vi "csv-from-string-timestamps.vi"(7 "LabVIEW Web Service Request":refnum<class "Web Request.lvclass">, 9 "format":string, 10 "end":string, 11 "start":string) -> (3 "Data":string)   [LabVIEW 2017]
uses:
  <vilib>/wsapi/Web Request.lvclass
  private/GlobalVariable.vi
panel:
  # "Use the Web Service Request input terminal to call the VIs on the Web Services palette. Do not remove it from the connector pane unless you don't need access to the palette."
  # "Each additional control wired to the connector pane will be available as an input in the URL. To include an indicator in terminal-mode output (the default setting), it must also be wired to the connector pane."
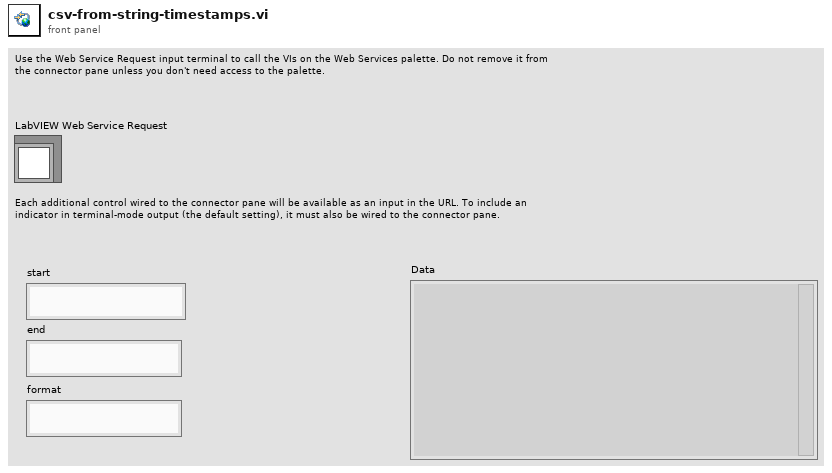
[diagram p1: front panel]
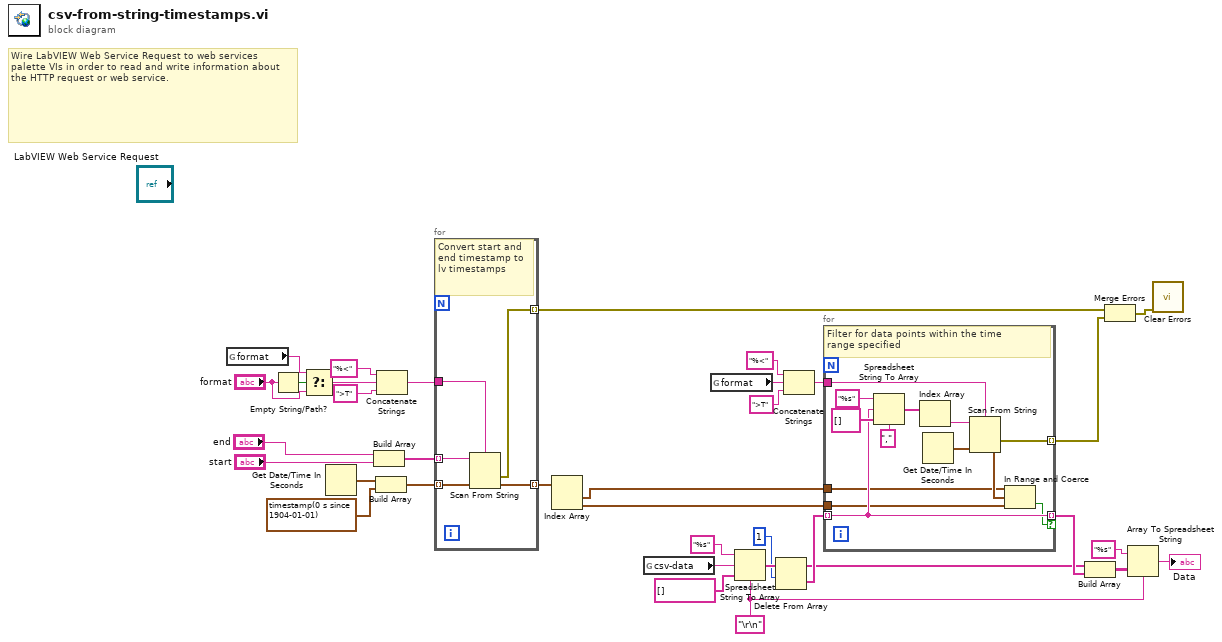
[diagram p0: block diagram]
diagram:
  w9 = "\r\n" ("format string")
  # "Wire LabVIEW Web Service Request to web services palette VIs in order to read and write information about the HTTP request or web service."
  n1 = global read "GlobalVariable.vi" "format"() -> (w4:string)
  n2 = Empty String/Path?(string/path="format") -> (empty?=w7:bool)
  n3 = Select(t=w4, s=w7, f="format") -> (s? t:f=w5:string)
  n4 = Get Date/Time In Seconds() -> (seconds since 1Jan1904=w31:timestamp)
  n5 = Build Array("end", "start") -> (w33:string[])
  n6 = Build Array(w31, timestamp(0 s since 1904-01-01) ("current time")) -> (w32:timestamp[])
  n7 = Concatenate Strings("%<" ("format string"), w5, ">T" ("input 2")) -> (w27:string)
  n8 = for {
    tunnel: w27 -> [w40]
    tunnel: w33 -> [w39] mode=indexing
    tunnel: w32 -> [w38] mode=indexing
    tunnel: [w37] -> w8 mode=indexing
    tunnel: [w36] -> w26 mode=indexing
    # "Convert start and end timestamp to lv timestamps"
    n9 = Scan From String(format string=w40, input string=w39, default 1=w38) -> (error out=w37:errorcluster, output 1=w36:timestamp)  [unwired: 2 in, 2 out]
  }
  n10 = Index Array(array=w26) -> (element #1=w10:timestamp, element #2=w11:timestamp)  [unwired: 2 in]
  n11 = global read "GlobalVariable.vi" "csv-data"() -> (w25:string)
  n12 = global read "GlobalVariable.vi" "format"() -> (w12:string)
  n13 = Spreadsheet String To Array(delimiter (Tab)=w9, format string="%s", spreadsheet string=w25, array type (2D Dbl)=string[] []) -> (array=w22:string[])
  n14 = Delete From Array(array=w22, length=1 ("index")) -> (deleted portion=w2:string[], array with subset deleted=w1:string[])  [unwired: 1 in]
  n15 = Concatenate Strings("%<" ("format string"), w12, ">T" ("input 2")) -> (w13:string)
  n16 = for {
    tunnel: w2 -> [w49] mode=indexing
    tunnel: [w49] -> w21 mode=indexing if=w43
    tunnel: [w47] -> w16 mode=indexing
    tunnel: w13 -> [w46]
    tunnel: w11 -> [w42]
    tunnel: w10 -> [w41]
    # "Filter for data points within the time \nrange specified"
    n17 = Spreadsheet String To Array(delimiter (Tab)="," ("format string"), format string="%s", spreadsheet string=w49, array type (2D Dbl)=string[] []) -> (array=w50:string[])
    n18 = Index Array(array=w50) -> (element=w48:string)  [unwired: 1 in]
    n19 = Get Date/Time In Seconds() -> (seconds since 1Jan1904=w45:timestamp)
    n20 = Scan From String(format string=w46, input string=w48, default 1=w45) -> (error out=w47:errorcluster, output 1=w44:timestamp)  [unwired: 2 in, 2 out]
    n21 = In Range and Coerce(upper limit=w41, x=w44, lower limit=w42) -> (In Range?=w43:bool)  [unwired: 1 out]
  }
  n22 = Build Array(w1, w21) -> (w20:string[][])
  n23 = Merge Errors(w8, w16) -> (w17:errorcluster)
  n24 = Array To Spreadsheet String(delimiter (Tab)=w9, array=w20, 3:"%s" ("format string")) -> (spreadsheet string=→"Data":string)
  n25 = call <vilib>:"Clear Errors.vi"("error in (no error)"=w17) -> ()  [unwired: 5 in, 2 out]
